vi "一体站流程自动启动.vi"(11 "参数":T1) -> ()   [LabVIEW 2016, in "PLC.lvlib"]
uses:
  PLC.lvlib
  <vilib>/ptbypt/NI_PtbyPt.lvlib
panel:
  out "s? t:f":enum16{"初始化", "采配水启动", "仪器操作", "反冲洗", "结束"}(ring)
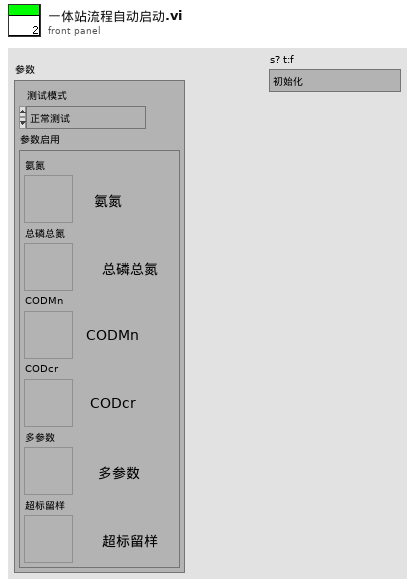
[diagram p1: front panel]
types:
  T1 = cluster{"测试模式":enum16{"正常测试", "集成干预"}, "参数启用":cluster{"氨氮":bool, "总磷总氮":bool, "CODMn":bool, "CODcr":bool, "多参数":bool, "超标留样":bool}}
  T2 = cluster{"命令":string, cluster{"starting address":u16, "holding register value":u16}}
  T3 = enum16{"启动测量", "标样核查", "零点核查", "跨度核查", "空白测试", "平行样测试", "加标回收", "空白校准", "标样校准", "初始化（清洗）", "停止测试", "仪器重启", "校时", "模式设置", "测量间隔设置"}
  T4 = cluster{"时间标识":timestamp, "设备":string, "日志信息":string, "流程参数":string}
  T5 = cluster{"测量模式":enum16{"水样测量", "标样核查", "零点核查", "跨度核查", "空白测试", "加标回收", "平行样", "校零", "校标"}}
  T6 = cluster{"时间标识":timestamp, "设备":string, "日志信息":string}
  T7 = enum16{"空闲", "水样测试", "标样核查", "零点核查", "跨度核查", "空白测试", "平行样测试", "加标回收", "空白校准", "标样校准", "初始化（清洗）"}
  T8 = enum32{"Bad", "Idle", "Run top level", "Running"}
  T9 = cluster{"R0":i16, "R1":i16, "R2":i16, "R3":i16, "R4":i16, "R5":i16, "R6":i16, "R7":i16, "R8":i16, "R9":i16, "R10":i16, "R11":i16, "R12":i16, "R13":i16, "R14":i16, "R15":i16, "R16":i16, "R17":i16, "R18":i16, "R19":i16, "R20":i16, "R21":i16, "R22":i16, "R23":i16, "R24":i16, "R25":i16, "R26":i16, "R27":i16, "R28":i16, "R29":i16, "R30":i16, "R31":i16, "R32":i16, "R33":i16, "R34":i16}
  T10 = cluster{"R100":i16, "R101":i16, "R102":i16, "R103":i16, "R104":i16, "R105":i16, "R106":i16, "R107":i16, "R108":i16, "R109":i16, "R110":i16, "R111":i16, "R112":i16, "R113":i16, "R114":i16, "R115":i16, "R116":i16, "R117":i16, "R118":i16, "R119":i16}
  T11 = cluster{"氨氮":bool, "总磷总氮":bool, "CODmn":bool, "CODCr":bool, "多参数":bool, "超标留样":bool}
  T12 = cluster{"因子编码":u32, "单位":u16, "标样参考值":sgl, "水样数据时间":timestamp, "水样实测值":sgl, "水样数据标识":string, "标样数据时间":timestamp, "标样实测值":sgl, "标样数据标识":string, "空白数据时间":timestamp, "空白实测值":sgl, "空白数据标识":string, "零点核查数据时间":timestamp, "零点核查实测值":sgl, "零点核查数据标识":string, "跨度核查数据时间":timestamp, "跨度核查实测值":sgl, "跨度核查数据标识":string, "加标回收数据时间":timestamp, "加标回收实测值":sgl, "加标回收数据标识":string, "平行样数据时间":timestamp, "平行样实测值":sgl, "平行样数据标识":string, "F0":sgl, "F1":sgl, "F2":sgl, "F3":sgl, "F4":sgl, "F5":sgl, "F6":sgl, "F7":sgl, "温度":sgl, "湿度":sgl, "X值":sgl, "fidrange":u16}
  T13 = cluster{"COD浓度（mg/L)":dbl, "水样启动时间":timestamp, "加标回收启动时间":timestamp, "CODMn工作状态":enum16{"空闲", "水样测试", "标样核查", "零点核查", "跨度核查", "空白测试", "平行样测试", "加标回收", "空白校准", "标样校准", "初始化（清洗）"}, "多列列表框":i32}
  T14 = cluster{"因子编码":u32, "单位":u16, "标样参考值":sgl, "水样数据时间":timestamp, "水样实测值":sgl, "水样数据标识":string, "标样数据时间":timestamp, "标样实测值":sgl, "标样数据标识":string, "空白数据时间":timestamp, "空白实测值":sgl, "空白数据标识":string, "零点核查数据时间":timestamp, "零点核查实测值":sgl, "零点核查数据标识":string, "跨度核查数据时间":timestamp, "跨度核查实测值":sgl, "跨度核查数据标识":string, "加标回收数据时间":timestamp, "加标回收实测值":sgl, "加标回收数据标识":string, "平行样数据时间":timestamp, "平行样实测值":sgl, "平行样数据标识":string}
  T15 = cluster{"氨氮":bool, "总磷总氮":bool, "CODMn":bool, "CODcr":bool, "多参数":bool, "超标留样":bool}
  T16 = cluster{"时间标识":timestamp, "参数":string, "数据类型":string, "集成干预测试浓度值":dbl, "集成干预前测试时间":timestamp, "集成干预前测试浓度值":dbl}
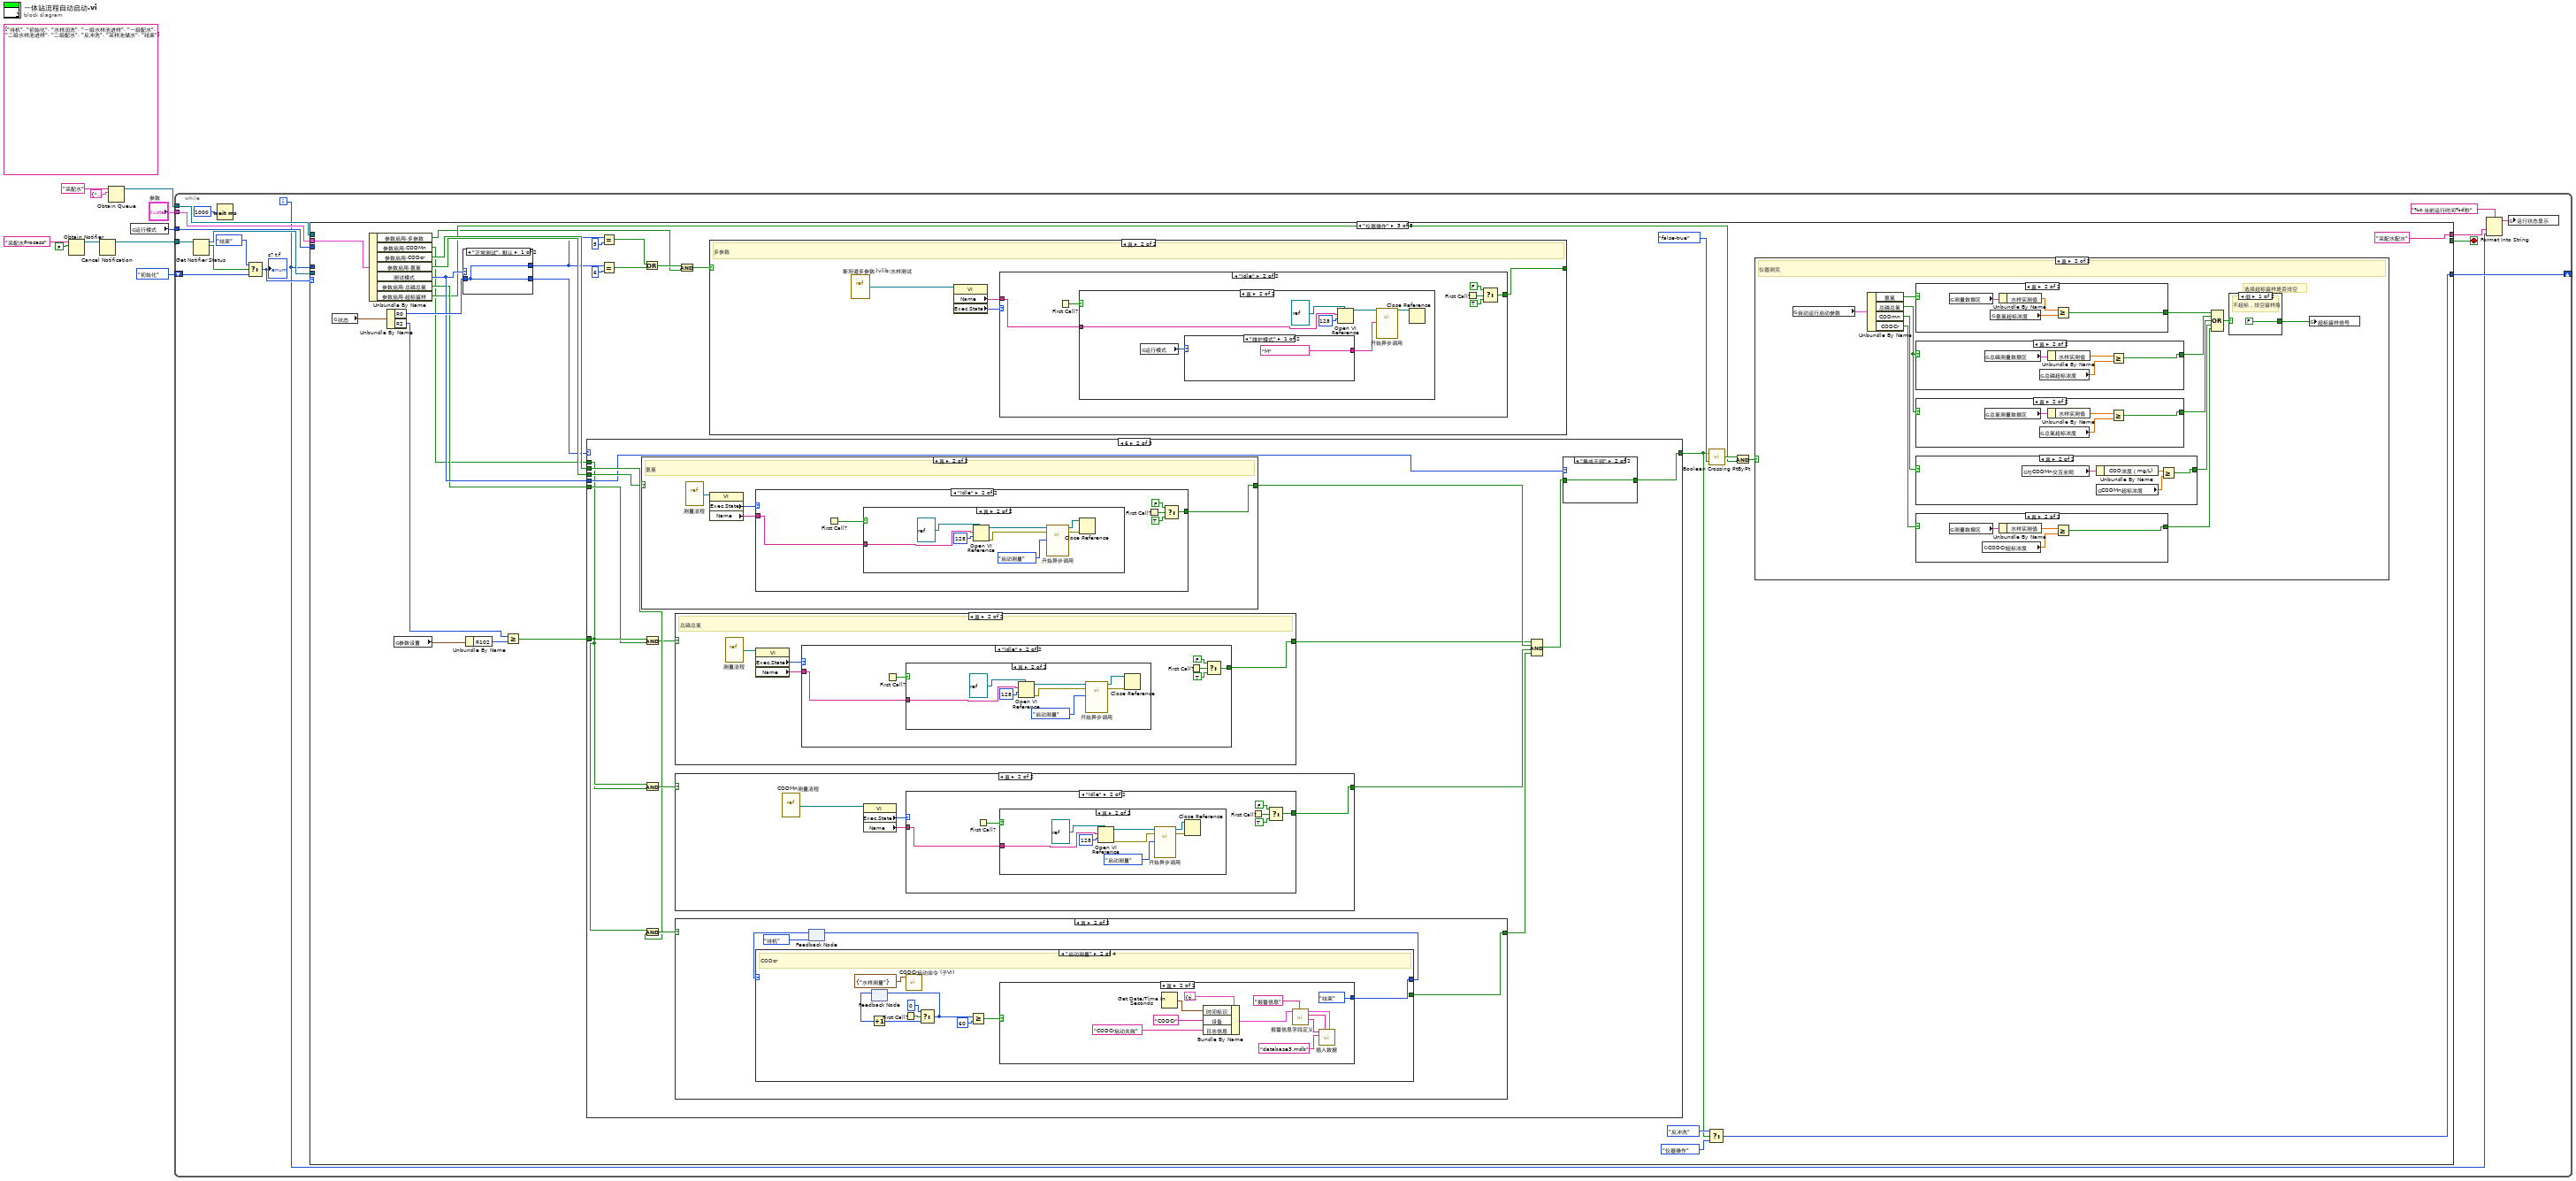
[diagram p0: block diagram]
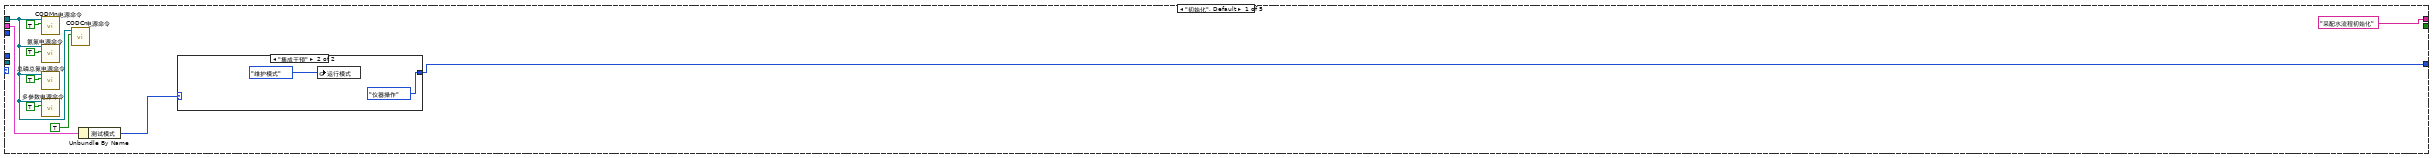
[diagram p2: hidden frame]
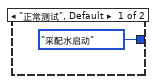
[diagram p3: hidden frame]
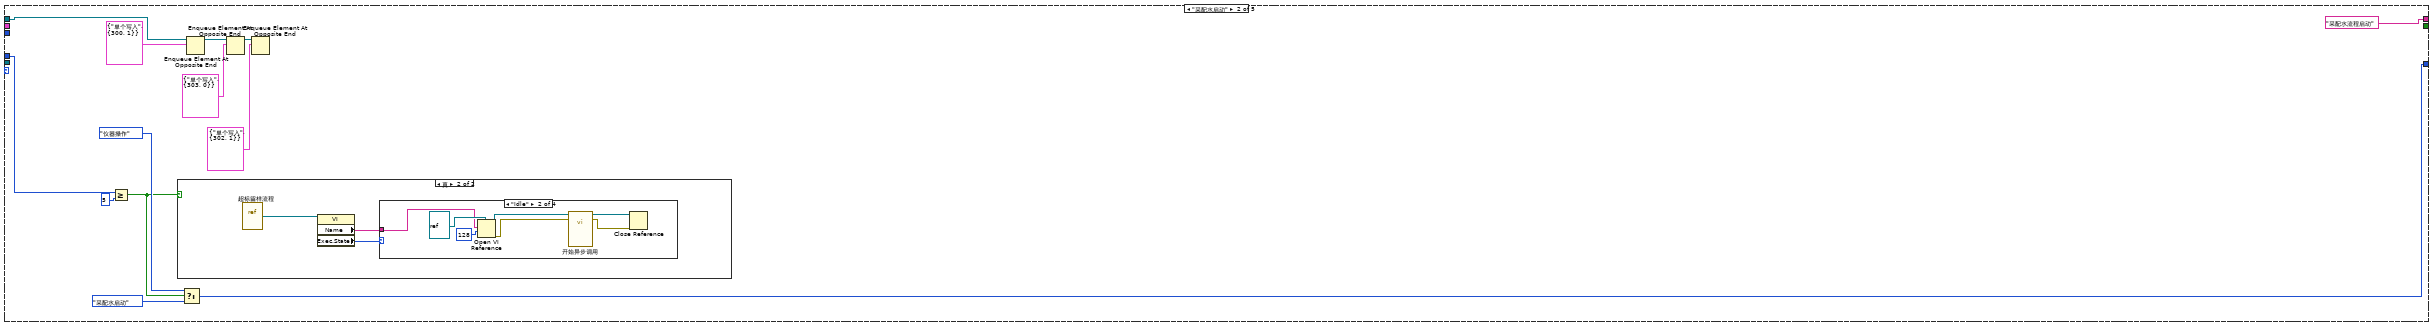
[diagram p4: hidden frame]
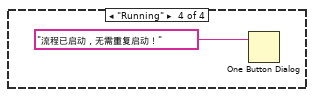
[diagram p8: hidden frame]
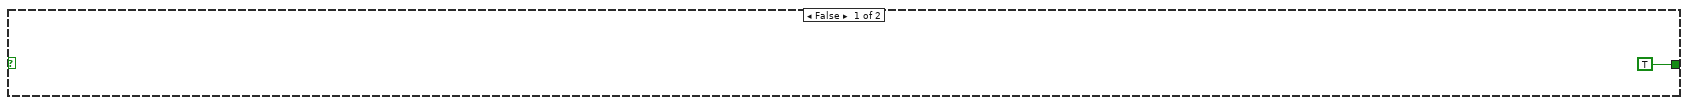
[diagram p9: hidden frame]
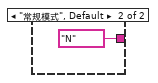
[diagram p12: hidden frame]
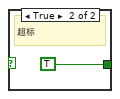
[diagram p14: hidden frame]
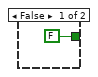
[diagram p15: hidden frame]
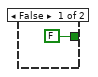
[diagram p16: hidden frame]
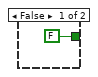
[diagram p17: hidden frame]
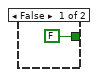
[diagram p18: hidden frame]
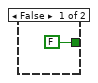
[diagram p19: hidden frame]
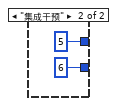
[diagram p20: hidden frame]
diagram:
  (unwired) string[][] [["待机"], ["初始化"], ["水样润洗"], ["一级水样池进样"], ["一级配水"], ["二级水样池进样"], ["二级配水"], ["反冲洗"], ["采样池储水"], ["结束"]] ("项名")
  n1 = Obtain Notifier(name (unnamed)="采配水Process" ("名称（未命名）"), notification data type=FALSE) -> (notifier out=w4:refnum<notifier>)  [unwired: 2 in, 2 out]
  n2 = Cancel Notification(0:w4) -> (8:w3:refnum<notifier>)  [unwired: 1 in, 2 out]
  n3 = Obtain Queue(name (unnamed)="采配水" ("名称（未命名）"), element data type=cluster{"命令":string, "数据":variant} {"命令"="", "数据"=variant}) -> (queue out=w7:refnum<queue>)  [unwired: 3 in, 2 out]
  n4 = global read "系统设置全局变量.vi" "运行模式"() -> (w1:enum16{"维护模式", "常规模式", "应急模式", "质控模式"})
  n5 = while {
    shift-right: [w23] -> _
    shift-left: enum16{"初始化", "采配水启动", "仪器操作", "反冲洗", "结束"}."初始化" ("枚举") -> [w19]
    tunnel: w7 -> [w26]
    tunnel: w3 -> [w22]
    tunnel: "参数" -> [w13]
    tunnel: w1 -> [w12]
    i -> [w11]
    stop <- w25 stop-if-true
    n6 = Get Notifier Status(notifier=w22) -> (notifier out=w14:refnum<notifier>, current notification=w21:bool)  [unwired: 1 in, 3 out]
    n7 = Wait (ms)(milliseconds to wait=u32 1000 ("等待时间（毫秒）")) -> ()  [unwired: 1 out]
    n8 = Select(t=enum16{"初始化", "采配水启动", "仪器操作", "反冲洗", "结束"}."结束" ("枚举"), s=w21, f=w19) -> (s? t:f=w18:enum16{"初始化", "采配水启动", "仪器操作", "反冲洗", "结束"})
    "s? t:f" <- w18
    n9 = case shown="\"仪器操作\"" w18 {
      tunnel: w26 -> [w31 w52 _ _ w475]
      tunnel: [_ _ _ _ TRUE] -> w25
      tunnel: [w30 w45 w89 w293 enum16{"初始化", "采配水启动", "仪器操作", "反冲洗", "结束"}."结束" ("枚举")] -> w23
      tunnel: ["采配水流程初始化" "采配水流程启动" "采配水配水" "等待测试完成" "采配水结束"] -> w15
      tunnel: w14 -> [_ _ _ _ w481]
      tunnel: w13 -> [w28 _ w91 w292 w478]
      tunnel: w12 -> [_ _ _ w289 w477]
      tunnel: w11 -> [_ w50 _ _ _]
      frame "初始化", Default {
        n10 = call "CODMn电源命令.vi"("通电/断电"=TRUE, "队列"=w31) -> ()  [unwired: 9 in, 1 out]
        n11 = call "氨氮电源命令.vi"("通电/断电"=TRUE, "队列"=w31) -> ()  [unwired: 9 in, 1 out]
        n12 = call "总磷总氮电源命令.vi"("通电/断电"=TRUE, "队列"=w31) -> ()  [unwired: 9 in, 1 out]
        n13 = call "多参数电源命令.vi"("通电/断电"=TRUE, "队列"=w31) -> ()  [unwired: 9 in, 1 out]
        n14 = call "CODCr电源命令.vi"("通电/断电"=TRUE, "队列"=w31) -> ()  [unwired: 9 in, 1 out]
        n15 = Unbundle By Name(w28) -> ("测试模式"=w27:enum16{"正常测试", "集成干预"})
        n16 = case shown="\"集成干预\"" w27 {
          tunnel: [enum16{"初始化", "采配水启动", "仪器操作", "反冲洗", "结束"}."采配水启动" ("枚举") enum16{"初始化", "采配水启动", "仪器操作", "反冲洗", "结束"}."仪器操作" ("枚举")] -> w30
          frame "正常测试", Default {
          }
          frame "集成干预" {
            n17 = global write "系统设置全局变量.vi" "运行模式"(enum16{"维护模式", "常规模式", "应急模式", "质控模式"}."维护模式" ("运行模式")) -> ()
          }
        }
      }
      frame "采配水启动" {
        n18 = Greater Or Equal?(x=w50, y=5) -> (x >= y?=w42:bool)
        n19 = case shown="真" w42 {
          frame False {
          }
          frame True {
            n20 = vi-ref "超标留样流程.vi"() -> (w55:refnum<vi>)
            n21 = property class="VI"(reference=w55) -> ("Name"=w54:string, "Exec.State"=w53:T8)  [unwired: 1 in, 2 out]
            n22 = case shown="\"Idle\"" w53 {
              tunnel: w54 -> [_ w58 _ _]
              frame "Bad", Default {
              }
              frame "Idle" {
                n23 = Open VI Reference(type specifier VI Refnum (for type only)=refnum<vi> refnum ("类型说明符VI引用句柄（仅用于类型）"), vi path=w58, options=128 ("选项")) -> (vi reference=w62:refnum<vi>, error out=w57:errorcluster)  [unwired: 3 in]
                n24 = call-by-ref "开始异步调用"(reference=w62, error in=w57) -> (reference out=w61:refnum<vi>, error out=w56:errorcluster)  [unwired: 12 in]
                n25 = Close Reference(reference=w61, error in (no error)=w56) -> ()  [unwired: 1 out]
              }
              frame "Run top level" {
              }
              frame "Running" {
                n26 = One Button Dialog(message="流程已启动，无需重复启动！" ("消息")) -> ()  [unwired: 1 in, 1 out]
              }
            }
          }
        }
        n27 = Select(t=enum16{"初始化", "采配水启动", "仪器操作", "反冲洗", "结束"}."仪器操作" ("枚举"), s=w42, f=enum16{"初始化", "采配水启动", "仪器操作", "反冲洗", "结束"}."采配水启动" ("枚举")) -> (s? t:f=w45:enum16{"初始化", "采配水启动", "仪器操作", "反冲洗", "结束"})
        n28 = Enqueue Element At Opposite End(queue=w52, element=T2 {"命令"="单个写入", {"starting address"=300, "holding register value"=1}} ("元素")) -> (queue out=w43:refnum<queue>)  [unwired: 2 in, 2 out]
        n29 = Enqueue Element At Opposite End(queue=w43, element=T2 {"命令"="单个写入", {"starting address"=303, "holding register value"=0}} ("元素")) -> (queue out=w40:refnum<queue>)  [unwired: 2 in, 2 out]
        n30 = Enqueue Element At Opposite End(queue=w40, element=T2 {"命令"="单个写入", {"starting address"=302, "holding register value"=1}} ("元素")) -> ()  [unwired: 2 in, 3 out]
      }
      frame "仪器操作" {
        n31 = global read "采配水全局变量.vi" "状态"() -> (w93:T9)
        n32 = Unbundle By Name(w91) -> ("参数启用.多参数"=w64:bool, "参数启用.CODMn"=w65:bool, "参数启用.CODcr"=w87:bool, "参数启用.氨氮"=w86:bool, "测试模式"=w79:enum16{"正常测试", "集成干预"}, "参数启用.总磷总氮"=w78:bool, "参数启用.超标留样"=w73:bool)
        n33 = Unbundle By Name(w93) -> ("R0"=w85:i16, "R2"=w80:i16)
        n34 = global read "采配水全局变量.vi" "参数设置"() -> (w82:T10)
        n35 = case shown="\"正常测试\", 默认" w79 {
          tunnel: w85 -> [w153 _]
          tunnel: [w153 i16 6 ("R0")] -> w84
          tunnel: [w153 i16 5 ("R0")] -> w70
          frame "正常测试", Default {
          }
          frame "集成干预" {
          }
        }
        n36 = Unbundle By Name(w82) -> ("R102"=w83:i16)
        n37 = Greater Or Equal?(x=w80, y=w83) -> (x >= y?=w81:bool)
        n38 = case shown="6" w84 {
          tunnel: [w157 w168 TRUE] -> w74
          tunnel: w87 -> [_ w175 _]
          tunnel: w86 -> [_ w174 _]
          tunnel: w81 -> [_ w167 _]
          tunnel: w79 -> [_ w170 _]
          tunnel: w78 -> [_ w166 _]
          tunnel: w65 -> [_ w163 _]
          frame 0, Default {
            n39 = global read "采配水全局变量.vi" "状态"() -> (w160:T9)
            n40 = global read "采配水全局变量.vi" "报警簇"() -> (w161:bool[])
            n41 = Unbundle By Name(w160) -> ("R0"=w159:i16)
            n42 = Equal To 0?(x=w159) -> (x = 0?=w162:bool)
            n43 = Index Array(array=w161, index=0 ("索引")) -> (element=w156:bool)
            n44 = Compound Arithmetic op=OR ("复合运算")(w162, w156) -> (w157:bool)
          }
          frame 6 {
            n45 = case "条件结构" shown="真" w174 {
              tunnel: [TRUE ("t") w199] -> w173
              frame False {
              }
              frame True {
                # "氨氮"
                n46 = vi-ref "测量流程.vi"() -> (w202:refnum<vi>)
                n47 = property class="VI"(reference=w202) -> ("Exec.State"=w201:T8, "Name"=w200:string)  [unwired: 1 in, 2 out]
                n48 = case shown="\"Idle\"" w201 {
                  tunnel: w200 -> [_ w208]
                  tunnel: [_ w203] -> w199
                  frame "Bad", Default {
                  }
                  frame "Idle" {
                    n49 = First Call?() -> (First Call?: T/F=w207:bool)
                    n50 = case shown="真" w207 {
                      tunnel: w208 -> [_ w213]
                      frame False {
                      }
                      frame True {
                        n51 = Open VI Reference(type specifier VI Refnum (for type only)=refnum<vi> refnum, vi path=w213, options=128 ("选项")) -> (vi reference=w211:refnum<vi>, error out=w214:errorcluster)  [unwired: 3 in]
                        n52 = call-by-ref "开始异步调用"(reference=w211, error in=w214, "控制命令"=T3."启动测量") -> (reference out=w215:refnum<vi>, error out=w216:errorcluster)  [unwired: 11 in]
                        n53 = Close Reference(reference=w215, error in (no error)=w216) -> ()  [unwired: 1 out]
                      }
                    }
                    n54 = First Call?() -> (First Call?: T/F=w206:bool)
                    n55 = Select(t=FALSE, s=w206, f=TRUE) -> (s? t:f=w203:bool)
                  }
                }
              }
            }
            n56 = And(x=w167, y=w166) -> (x .and. y?=w165:bool)
            n57 = And(x=w167, y=w163) -> (x .and. y?=w177:bool)
            n58 = And(x=w167, y=w175) -> (x .and. y?=w176:bool)
            n59 = case "条件结构" shown="真" w165 {
              tunnel: [TRUE ("t") w179] -> w164
              frame False {
              }
              frame True {
                # "总磷总氮"
                n60 = vi-ref "测量流程.vi"() -> (w182:refnum<vi>)
                n61 = property class="VI"(reference=w182) -> ("Exec.State"=w181:T8, "Name"=w180:string)  [unwired: 1 in, 2 out]
                n62 = case shown="\"Idle\"" w181 {
                  tunnel: w180 -> [_ w188]
                  tunnel: [_ w183] -> w179
                  frame "Bad", Default {
                  }
                  frame "Idle" {
                    n63 = First Call?() -> (First Call?: T/F=w187:bool)
                    n64 = case shown="真" w187 {
                      tunnel: w188 -> [_ w193]
                      frame False {
                      }
                      frame True {
                        n65 = Open VI Reference(type specifier VI Refnum (for type only)=refnum<vi> refnum, vi path=w193, options=128 ("选项")) -> (vi reference=w191:refnum<vi>, error out=w194:errorcluster)  [unwired: 3 in]
                        n66 = call-by-ref "开始异步调用"(reference=w191, error in=w194, "控制命令"=T3."启动测量") -> (reference out=w195:refnum<vi>, error out=w196:errorcluster)  [unwired: 11 in]
                        n67 = Close Reference(reference=w195, error in (no error)=w196) -> ()  [unwired: 1 out]
                      }
                    }
                    n68 = First Call?() -> (First Call?: T/F=w186:bool)
                    n69 = Select(t=FALSE, s=w186, f=TRUE) -> (s? t:f=w183:bool)
                  }
                }
              }
            }
            n70 = case shown="真" w177 {
              tunnel: [TRUE w270] -> w172
              frame False {
              }
              frame True {
                n71 = vi-ref "CODMn测量流程.vi"() -> (w271:refnum<vi>)
                n72 = property class="VI"(reference=w271) -> ("Exec.State"=w272:T8, "Name"=w273:string)  [unwired: 1 in, 2 out]
                n73 = case shown="\"Idle\"" w272 {
                  tunnel: w273 -> [_ w279]
                  tunnel: [_ w274] -> w270
                  frame "Bad", Default {
                  }
                  frame "Idle" {
                    n74 = First Call?() -> (First Call?: T/F=w278:bool)
                    n75 = case shown="真" w278 {
                      tunnel: w279 -> [_ w284]
                      frame False {
                      }
                      frame True {
                        n76 = Open VI Reference(type specifier VI Refnum (for type only)=refnum<vi> refnum, vi path=w284, options=128 ("选项")) -> (vi reference=w282:refnum<vi>, error out=w285:errorcluster)  [unwired: 3 in]
                        n77 = call-by-ref "开始异步调用"(reference=w282, error in=w285, "控制命令"=T3."启动测量") -> (reference out=w286:refnum<vi>, error out=w287:errorcluster)  [unwired: 11 in]
                        n78 = Close Reference(reference=w286, error in (no error)=w287) -> ()  [unwired: 1 out]
                      }
                    }
                    n79 = First Call?() -> (First Call?: T/F=w277:bool)
                    n80 = Select(t=FALSE, s=w277, f=TRUE) -> (s? t:f=w274:bool)
                  }
                }
              }
            }
            n81 = case shown="真" w176 {
              tunnel: [TRUE w218] -> w171
              frame False {
              }
              frame True {
                n82 = feedback #1(enum16{"待机", "启动测量", "测量中", "结束"}."待机") -> (w220:enum16{"待机", "启动测量", "测量中", "结束"})
                n83 = case shown="\"启动测量\"" w220 {
                  tunnel: [enum16{"待机", "启动测量", "测量中", "结束"}."启动测量" w236 w256 enum16{"待机", "启动测量", "测量中", "结束"}."结束"] -> w219
                  tunnel: [_ _ _ TRUE] -> w218
                  frame "待机", Default {
                    n84 = Get Date/Time In Seconds() -> (seconds since 1Jan1904=w226:timestamp)
                    n85 = Bundle By Name(cluster=T4 {"时间标识"=timestamp(0 s since 1904-01-01), "设备"="", "日志信息"="", "流程参数"=""} ("data in"), "时间标识"=w226, "设备"="CODCr", "日志信息"="-->>CODCr启动") -> (w222:T4)
                    n86 = call "总磷总氮操作日志.vi"("data in"=w222) -> ()  [unwired: 11 in]
                  }
                  frame "启动测量" {
                    # "CODcr"
                    n87 = feedback #2() -> (w232:i32)  [unwired: 1 in]
                    n88 = Increment(x=w232) -> (x+1=w233:i32)
                    n89 = First Call?() -> (First Call?: T/F=w231:bool)
                    n90 = call "CODCr启动命令 (子VI).vi"("启动测量模式"=T5 {"测量模式"=enum."水样测量"}) -> ()  [unwired: 11 in]
                    n91 = Select(t=0, s=w231, f=w233) -> (s? t:f=w234:i32)
                    n92 = feedback-in #2(w234) -> ()
                    n93 = Greater Or Equal?(x=w234, y=60) -> (x >= y?=w229:bool)
                    n94 = case shown="真" w229 {
                      tunnel: [w237 enum16{"待机", "启动测量", "测量中", "结束"}."结束"] -> w236
                      frame False {
                        n95 = global read "CODcr全局变量.vi" "工作状态"() -> (w238:T7)
                        n96 = Not Equal To 0?(x=w238) -> (x != 0?=w239:bool)
                        n97 = Select(t=enum16{"待机", "启动测量", "测量中", "结束"}."测量中", s=w239, f=enum16{"待机", "启动测量", "测量中", "结束"}."启动测量") -> (s? t:f=w237:enum16{"待机", "启动测量", "测量中", "结束"})
                      }
                      frame True {
                        n98 = Get Date/Time In Seconds() -> (seconds since 1Jan1904=w248:timestamp)
                        n99 = Bundle By Name(cluster=T6 {"时间标识"=timestamp(0 s since 1904-01-01), "设备"="", "日志信息"=""} ("data in"), "时间标识"=w248, "设备"="CODCr", "日志信息"="CODCr启动失败") -> (w242:T6)
                        n100 = call "报警信息字段定义.vi"("table输入"="报警信息", "data in"=w242) -> ("table输出"=w245:string, "columns"=w246:string[], "data out"=w247:T6)  [unwired: 7 in]
                        n101 = call "插入数据.vi"("data"=w247, "columns"=w246, "database"="database3.mdb", "table"=w245) -> ()  [unwired: 7 in, 1 out]
                      }
                    }
                  }
                  frame "测量中" {
                    n102 = global read "CODcr全局变量.vi" "工作状态"() -> (w255:T7)
                    n103 = Equal?(x=w255, y=T7."空闲" ("工作状态")) -> (x = y?=w254:bool)
                    n104 = case shown="假" w254 {
                      tunnel: [w257 enum16{"待机", "启动测量", "测量中", "结束"}."结束"] -> w256
                      frame False {
                        n105 = flat-sequence {
                          tunnel: [enum16{"待机", "启动测量", "测量中", "结束"}."测量中"] -> w257
                          frame #0 {
                            n106 = Wait (ms)(milliseconds to wait=u32 1000 ("等待时间（毫秒）")) -> ()  [unwired: 1 out]
                          }
                          frame #1 {
                          }
                        }
                      }
                      frame True {
                      }
                    }
                  }
                  frame "结束" {
                    n107 = First Call?() -> (First Call?: T/F=w261:bool)
                    n108 = case shown="真" w261 {
                      frame False {
                      }
                      frame True {
                        n109 = Get Date/Time In Seconds() -> (seconds since 1Jan1904=w268:timestamp)
                        n110 = Bundle By Name(cluster=T4 {"时间标识"=timestamp(0 s since 1904-01-01), "设备"="", "日志信息"="", "流程参数"=""} ("data in"), "时间标识"=w268, "设备"="CODCr", "日志信息"="-->>CODCr停止") -> (w264:T4)
                        n111 = call "总磷总氮操作日志.vi"("data in"=w264) -> ()  [unwired: 11 in]
                      }
                    }
                  }
                }
                n112 = feedback-in #1(w219) -> ()
              }
            }
            n113 = Compound Arithmetic op=AND ("复合运算")(w164, w173, w172, w171) -> (w169:bool)
            n114 = case shown="\"集成干预\"" w170 {
              tunnel: w169 -> [_ w197]
              tunnel: [_ w197] -> w168
              frame "正常测试", Default {
              }
              frame "集成干预" {
              }
            }
          }
          frame 7..9 {
          }
        }
        n115 = Equal?(x=w70, y=i16 5) -> (x = y?=w71:bool)
        n116 = Equal?(x=w70, y=i16 6) -> (x = y?=w67:bool)
        n117 = Or(x=w71, y=w67) -> (x .or. y?=w68:bool)
        n118 = And(x=w68, y=w64) -> (x .and. y?=w66:bool)
        n119 = case shown="真" w66 {
          tunnel: [TRUE ("t") w95] -> _
          frame False {
          }
          frame True {
            # "多参数"
            n120 = vi-ref "斯坦道多参数.lvlib:水样测试.vi"() -> (w97:refnum<vi>)
            n121 = property class="VI"(reference=w97) -> ("Name"=w96:string, "Exec.State"=w98:T8)  [unwired: 1 in, 2 out]
            n122 = case shown="\"Idle\"" w98 {
              tunnel: w96 -> [_ w104]
              tunnel: [_ w99] -> w95
              frame "Bad", Default {
              }
              frame "Idle" {
                n123 = First Call?() -> (First Call?: T/F=w103:bool)
                n124 = case shown="真" w103 {
                  tunnel: w104 -> [_ w110]
                  frame False {
                  }
                  frame True {
                    n125 = global read "系统设置全局变量.vi" "运行模式"() -> (w107:enum16{"维护模式", "常规模式", "应急模式", "质控模式"})
                    n126 = case shown="\"维护模式\"" w107 {
                      tunnel: ["M" ("数据标记表") "N" ("数据标记表")] -> w106
                      frame "维护模式" {
                      }
                      frame "常规模式", Default {
                      }
                    }
                    n127 = Open VI Reference(type specifier VI Refnum (for type only)=refnum<vi> refnum, vi path=w110, options=128 ("选项")) -> (vi reference=w109:refnum<vi>)  [unwired: 3 in, 1 out]
                    n128 = call-by-ref "开始异步调用"(reference=w109, "数据标记表"=w106) -> (reference out=w108:refnum<vi>)  [unwired: 12 in, 1 out]
                    n129 = Close Reference(reference=w108) -> ()  [unwired: 1 in, 1 out]
                  }
                }
                n130 = First Call?() -> (First Call?: T/F=w102:bool)
                n131 = Select(t=FALSE, s=w102, f=TRUE) -> (s? t:f=w99:bool)
              }
            }
          }
        }
        n132 = Select(t=enum16{"初始化", "采配水启动", "仪器操作", "反冲洗", "结束"}."反冲洗" ("枚举"), s=w74, f=enum16{"初始化", "采配水启动", "仪器操作", "反冲洗", "结束"}."仪器操作" ("枚举")) -> (s? t:f=w89:enum16{"初始化", "采配水启动", "仪器操作", "反冲洗", "结束"})
        n133 = call <vilib>:"Boolean Crossing PtByPt.vi"("direction"=enum16{"either", "false-true", "true-false"}."false-true", "input"=w74) -> ("crossing"=w76:bool)  [unwired: 1 in]
        n134 = And(x=w76, y=w73) -> (x .and. y?=w75:bool)
        n135 = case shown="真" w75 {
          frame False {
          }
          frame True {
            # "选择超标留样是否排空"
            # "仪器测完"
            n136 = global read "系统设置全局变量.vi" "自动运行启动参数"() -> (w118:T11)
            n137 = Unbundle By Name(w118) -> ("氨氮"=w117:bool, "总磷总氮"=w116:bool, "CODmn"=w115:bool, "CODCr"=w114:bool)
            n138 = case shown="真" w117 {
              tunnel: [FALSE w151] -> w125
              frame False {
              }
              frame True {
                n139 = global read "VAR总磷总氮全局变量.vi" "测量数据区"() -> (w150:T12)
                n140 = global read "外部交互全局.vi" "氨氮超标浓度"() -> (w149:dbl)
                n141 = Unbundle By Name(w150) -> ("水样实测值"=w152:sgl)
                n142 = Greater Or Equal?(x=w152, y=w149) -> (x >= y?=w151:bool)
              }
            }
            n143 = case shown="真" w116 {
              tunnel: [FALSE w147] -> w124
              frame False {
              }
              frame True {
                n144 = global read "VAR总磷总氮全局变量.vi" "总磷测量数据区"() -> (w144:T12)
                n145 = global read "外部交互全局.vi" "总磷超标浓度"() -> (w145:dbl)
                n146 = Unbundle By Name(w144) -> ("水样实测值"=w146:sgl)
                n147 = Greater Or Equal?(x=w146, y=w145) -> (x >= y?=w147:bool)
              }
            }
            n148 = case shown="真" w116 {
              tunnel: [FALSE w142] -> w123
              frame False {
              }
              frame True {
                n149 = global read "VAR总磷总氮全局变量.vi" "总氮测量数据区"() -> (w139:T12)
                n150 = global read "外部交互全局.vi" "总氮超标浓度"() -> (w140:dbl)
                n151 = Unbundle By Name(w139) -> ("水样实测值"=w141:sgl)
                n152 = Greater Or Equal?(x=w141, y=w140) -> (x >= y?=w142:bool)
              }
            }
            n153 = case shown="真" w115 {
              tunnel: [FALSE w137] -> w122
              frame False {
              }
              frame True {
                n154 = global read "modbus slave全局.vi" "与CODMn交互全局"() -> (w135:T13)
                n155 = Unbundle By Name(w135) -> ("COD浓度（mg/L)"=w134:dbl)
                n156 = global read "外部交互全局.vi" "CODMn超标浓度"() -> (w136:dbl)
                n157 = Greater Or Equal?(x=w134, y=w136) -> (x >= y?=w137:bool)
              }
            }
            n158 = case shown="真" w114 {
              tunnel: [FALSE w132] -> w121
              frame False {
              }
              frame True {
                n159 = global read "CODcr全局变量.vi" "测量数据区"() -> (w129:T14)
                n160 = global read "外部交互全局.vi" "CODCr超标浓度"() -> (w130:dbl)
                n161 = Unbundle By Name(w129) -> ("水样实测值"=w131:sgl)
                n162 = Greater Or Equal?(x=w131, y=w130) -> (x >= y?=w132:bool)
              }
            }
            n163 = Compound Arithmetic op=OR ("复合运算")(w125, w124, w123, w122, w121) -> (w120:bool)
            n164 = case shown="假" w120 {
              tunnel: [FALSE ("超标留样信号") TRUE ("超标留样信号")] -> w119
              frame False {
                # "不超标，排空留样瓶"
              }
              frame True {
                # "超标"
              }
            }
            n165 = global write "外部交互全局.vi" "超标留样信号"(w119) -> ()
          }
        }
      }
      frame "反冲洗" {
        n166 = First Call?() -> (First Call?: T/F=w290:bool)
        n167 = case shown="真" w290 {
          tunnel: w292 -> [_ w302]
          tunnel: w289 -> [_ w299]
          frame False {
          }
          frame True {
            n168 = Unbundle By Name(w302) -> ("测试模式"=w301:enum16{"正常测试", "集成干预"}, "参数启用"=w300:T15)
            n169 = case shown="\"正常测试\", 默认" w301 {
              tunnel: w300 -> [w311 w398]
              tunnel: w299 -> [_ w392]
              frame "正常测试", Default {
                n170 = global read "系统设置全局变量.vi" "运行模式"() -> (w309:enum16{"维护模式", "常规模式", "应急模式", "质控模式"})
                n171 = global read "采配水全局变量.vi" "输入状态"() -> (w308:bool[])
                n172 = global read "采配水全局变量.vi" "报警簇"() -> (w316:bool[])
                n173 = case shown="\"维护模式\"" w309 {
                  tunnel: ["M" ("table") "N" ("table")] -> w310
                  frame "维护模式" {
                  }
                  frame "常规模式", Default {
                  }
                }
                n174 = Index Array(array=w308, index=7 ("索引")) -> (element=w306:bool)
                n175 = Index Array(array=w316, index #1=0 ("索引"), index #2=11 ("索引")) -> (element #1=w313:bool, element #2=w312:bool)
                n176 = Select(t="P" ("数据标识"), s=w306, f="Z" ("数据标识")) -> (s? t:f=w303:string)
                n177 = case shown="真" w313 {
                  tunnel: w312 -> [w322 _]
                  tunnel: w311 -> [w321 w336]
                  tunnel: w310 -> [w319 w330]
                  tunnel: w303 -> [_ w329]
                  frame False {
                    n178 = Unbundle By Name(w321) -> ("氨氮"=w320:bool)
                    n179 = case shown="真" w322 {
                      tunnel: w320 -> [_ w324]
                      tunnel: w319 -> [_ w323]
                      frame False {
                      }
                      frame True {
                        n180 = case shown="真" w324 {
                          tunnel: w323 -> [_ w325]
                          tunnel: [_ w326] -> _
                          frame False {
                          }
                          frame True {
                            n181 = call "取水点无水样数据存储.vi"("数据标识"="lw", "数据类型"=w325, "table"="氨氮") -> ("error out"=w326:errorcluster)  [unwired: 8 in]
                          }
                        }
                      }
                    }
                  }
                  frame True {
                    n182 = Unbundle By Name(w336) -> ("氨氮"=w335:bool, "CODMn"=w334:bool, "CODcr"=w333:bool, "多参数"=w332:bool, "总磷总氮"=w331:bool)
                    n183 = case shown="真" w335 {
                      tunnel: w330 -> [_ w389]
                      tunnel: [_ w390] -> _
                      tunnel: w329 -> [_ w388]
                      frame False {
                      }
                      frame True {
                        n184 = call "取水点无水样数据存储.vi"("数据标识"=w388, "数据类型"=w389, "table"="氨氮") -> ("error out"=w390:errorcluster)  [unwired: 8 in]
                      }
                    }
                    n185 = case shown="真" w334 {
                      tunnel: w330 -> [_ w386]
                      tunnel: [_ w385] -> _
                      tunnel: w329 -> [_ w384]
                      frame False {
                      }
                      frame True {
                        n186 = call "取水点无水样数据存储.vi"("数据标识"=w384, "数据类型"=w386, "table"="CODMn") -> ("error out"=w385:errorcluster)  [unwired: 8 in]
                      }
                    }
                    n187 = case shown="真" w333 {
                      tunnel: w330 -> [_ w382]
                      tunnel: [_ w381] -> _
                      tunnel: w329 -> [_ w380]
                      frame False {
                      }
                      frame True {
                        n188 = call "取水点无水样数据存储.vi"("数据标识"=w380, "数据类型"=w382, "table"="CODCr") -> ("error out"=w381:errorcluster)  [unwired: 8 in]
                      }
                    }
                    n189 = case shown="真" w331 {
                      tunnel: w330 -> [_ w337]
                      tunnel: [_ w339] -> _
                      tunnel: w329 -> [_ w338]
                      frame False {
                      }
                      frame True {
                        n190 = call "取水点无水样数据存储.vi"("数据标识"=w338, "数据类型"=w337, "table"="总氮") -> ("error out"=w340:errorcluster)  [unwired: 8 in]
                        n191 = call "取水点无水样数据存储.vi"("error in (no error)"=w340, "数据标识"=w337, "数据类型"=w337, "table"="总磷") -> ("error out"=w339:errorcluster)  [unwired: 7 in]
                      }
                    }
                    n192 = case shown="真" w332 {
                      tunnel: w330 -> [_ w351]
                      tunnel: w329 -> [_ w343]
                      frame False {
                      }
                      frame True {
                        n193 = global read "断电保存变量.vi" "Cond"() -> (w346:bool)
                        n194 = global read "断电保存变量.vi" "Turb"() -> (w347:bool)
                        n195 = global read "断电保存变量.vi" "DO"() -> (w348:bool)
                        n196 = global read "断电保存变量.vi" "pH"() -> (w349:bool)
                        n197 = case shown="真" w349 {
                          tunnel: w351 -> [_ w374]
                          tunnel: [_ w373] -> _
                          tunnel: w343 -> [_ w372]
                          frame False {
                          }
                          frame True {
                            n198 = call "取水点无水样数据存储.vi"("数据标识"=w372, "数据类型"=w374, "table"="pH") -> ("error out"=w373:errorcluster)  [unwired: 8 in]
                          }
                        }
                        n199 = case shown="真" w348 {
                          tunnel: w351 -> [_ w370]
                          tunnel: [_ w369] -> _
                          tunnel: w343 -> [_ w368]
                          frame False {
                          }
                          frame True {
                            n200 = call "取水点无水样数据存储.vi"("数据标识"=w368, "数据类型"=w370, "table"="DO") -> ("error out"=w369:errorcluster)  [unwired: 8 in]
                          }
                        }
                        n201 = case shown="真" w347 {
                          tunnel: w351 -> [_ w362]
                          tunnel: [_ w361] -> _
                          tunnel: w343 -> [_ w360]
                          frame False {
                          }
                          frame True {
                            n202 = call "取水点无水样数据存储.vi"("数据标识"=w360, "数据类型"=w362, "table"="浊度") -> ("error out"=w361:errorcluster)  [unwired: 8 in]
                          }
                        }
                        n203 = case shown="真" w346 {
                          tunnel: w351 -> [_ w366]
                          tunnel: [_ w365] -> _
                          tunnel: w343 -> [_ w364]
                          frame False {
                          }
                          frame True {
                            n204 = call "取水点无水样数据存储.vi"("数据标识"=w364, "数据类型"=w366, "table"="电导率") -> ("error out"=w365:errorcluster)  [unwired: 8 in]
                          }
                        }
                        n205 = global read "断电保存变量.vi" "藻密度"() -> (w344:bool)
                        n206 = global read "断电保存变量.vi" "Temp"() -> (w350:bool)
                        n207 = global read "断电保存变量.vi" "叶绿素a启用"() -> (w345:bool)
                        n208 = case shown="真" w344 {
                          tunnel: w351 -> [_ w354]
                          tunnel: [_ w353] -> _
                          tunnel: w343 -> [_ w352]
                          frame False {
                          }
                          frame True {
                            n209 = call "取水点无水样数据存储.vi"("数据标识"=w352, "数据类型"=w354, "table"="藻密度") -> ("error out"=w353:errorcluster)  [unwired: 8 in]
                          }
                        }
                        n210 = case shown="真" w350 {
                          tunnel: w351 -> [_ w378]
                          tunnel: [_ w377] -> _
                          tunnel: w343 -> [_ w376]
                          frame False {
                          }
                          frame True {
                            n211 = call "取水点无水样数据存储.vi"("数据标识"=w376, "数据类型"=w378, "table"="水温") -> ("error out"=w377:errorcluster)  [unwired: 8 in]
                          }
                        }
                        n212 = case shown="真" w345 {
                          tunnel: w351 -> [_ w358]
                          tunnel: [_ w357] -> _
                          tunnel: w343 -> [_ w356]
                          frame False {
                          }
                          frame True {
                            n213 = call "取水点无水样数据存储.vi"("数据标识"=w356, "数据类型"=w358, "table"="叶绿素a") -> ("error out"=w357:errorcluster)  [unwired: 8 in]
                          }
                        }
                      }
                    }
                  }
                }
              }
              frame "集成干预" {
                n214 = Unbundle By Name(w398) -> ("氨氮"=w397:bool, "CODMn"=w396:bool, "CODcr"=w395:bool, "多参数"=w394:bool, "总磷总氮"=w393:bool)
                n215 = case shown="真" w397 {
                  tunnel: w392 -> [_ w470]
                  frame False {
                  }
                  frame True {
                    n216 = call "获取最近两组水样测试数据.vi"("运行模式"=w470, "table"="氨氮") -> ("error out"=w471:errorcluster, "存储变量"=w472:T16)  [unwired: 8 in]
                    n217 = call "集成干预测试数据存储.vi"("error in (no error)"=w471, "存储变量"=w472) -> ()  [unwired: 9 in, 1 out]
                  }
                }
                n218 = case shown="真" w396 {
                  tunnel: w392 -> [_ w466]
                  frame False {
                  }
                  frame True {
                    n219 = call "获取最近两组水样测试数据.vi"("运行模式"=w466, "table"="CODMn") -> ("error out"=w467:errorcluster, "存储变量"=w468:T16)  [unwired: 8 in]
                    n220 = call "集成干预测试数据存储.vi"("error in (no error)"=w467, "存储变量"=w468) -> ()  [unwired: 9 in, 1 out]
                  }
                }
                n221 = case shown="真" w395 {
                  tunnel: w392 -> [_ w462]
                  frame False {
                  }
                  frame True {
                    n222 = call "获取最近两组水样测试数据.vi"("运行模式"=w462, "table"="CODCr") -> ("error out"=w463:errorcluster, "存储变量"=w464:T16)  [unwired: 8 in]
                    n223 = call "集成干预测试数据存储.vi"("error in (no error)"=w463, "存储变量"=w464) -> ()  [unwired: 9 in, 1 out]
                  }
                }
                n224 = case shown="真" w393 {
                  tunnel: w392 -> [_ w399]
                  frame False {
                  }
                  frame True {
                    n225 = call "获取最近两组水样测试数据.vi"("运行模式"=w399, "table"="总磷") -> ("error out"=w404:errorcluster, "存储变量"=w405:T16)  [unwired: 8 in]
                    n226 = call "集成干预测试数据存储.vi"("error in (no error)"=w404, "存储变量"=w405) -> ("error out"=w400:errorcluster)  [unwired: 9 in]
                    n227 = call "获取最近两组水样测试数据.vi"("error in (no error)"=w400, "运行模式"=w399, "table"="总氮") -> ("error out"=w403:errorcluster, "存储变量"=w402:T16)  [unwired: 7 in]
                    n228 = call "集成干预测试数据存储.vi"("error in (no error)"=w403, "存储变量"=w402) -> ()  [unwired: 9 in, 1 out]
                  }
                }
                n229 = case shown="真" w394 {
                  tunnel: w392 -> [_ w407]
                  frame False {
                  }
                  frame True {
                    n230 = global read "断电保存变量.vi" "Temp"() -> (w414:bool)
                    n231 = case shown="真" w414 {
                      tunnel: [_ w458] -> w420
                      tunnel: w407 -> [_ w457]
                      frame False {
                      }
                      frame True {
                        n232 = call "获取最近两组水样测试数据.vi"("运行模式"=w457, "table"="水温") -> ("error out"=w461:errorcluster, "存储变量"=w460:T16)  [unwired: 8 in]
                        n233 = call "集成干预测试数据存储.vi"("error in (no error)"=w461, "存储变量"=w460) -> ("error out"=w458:errorcluster)  [unwired: 9 in]
                      }
                    }
                    n234 = global read "断电保存变量.vi" "pH"() -> (w413:bool)
                    n235 = case shown="真" w413 {
                      tunnel: [_ w453] -> w419
                      tunnel: w420 -> [_ w452]
                      tunnel: w407 -> [_ w451]
                      frame False {
                      }
                      frame True {
                        n236 = call "获取最近两组水样测试数据.vi"("error in (no error)"=w452, "运行模式"=w451, "table"="pH") -> ("error out"=w456:errorcluster, "存储变量"=w455:T16)  [unwired: 7 in]
                        n237 = call "集成干预测试数据存储.vi"("error in (no error)"=w456, "存储变量"=w455) -> ("error out"=w453:errorcluster)  [unwired: 9 in]
                      }
                    }
                    n238 = global read "断电保存变量.vi" "DO"() -> (w412:bool)
                    n239 = case shown="真" w412 {
                      tunnel: [_ w447] -> w418
                      tunnel: w419 -> [_ w446]
                      tunnel: w407 -> [_ w445]
                      frame False {
                      }
                      frame True {
                        n240 = call "获取最近两组水样测试数据.vi"("error in (no error)"=w446, "运行模式"=w445, "table"="DO") -> ("error out"=w450:errorcluster, "存储变量"=w449:T16)  [unwired: 7 in]
                        n241 = call "集成干预测试数据存储.vi"("error in (no error)"=w450, "存储变量"=w449) -> ("error out"=w447:errorcluster)  [unwired: 9 in]
                      }
                    }
                    n242 = global read "断电保存变量.vi" "Cond"() -> (w411:bool)
                    n243 = case shown="真" w411 {
                      tunnel: [_ w441] -> w417
                      tunnel: w418 -> [_ w440]
                      tunnel: w407 -> [_ w439]
                      frame False {
                      }
                      frame True {
                        n244 = call "获取最近两组水样测试数据.vi"("error in (no error)"=w440, "运行模式"=w439, "table"="电导率") -> ("error out"=w444:errorcluster, "存储变量"=w443:T16)  [unwired: 7 in]
                        n245 = call "集成干预测试数据存储.vi"("error in (no error)"=w444, "存储变量"=w443) -> ("error out"=w441:errorcluster)  [unwired: 9 in]
                      }
                    }
                    n246 = global read "断电保存变量.vi" "Turb"() -> (w410:bool)
                    n247 = case shown="真" w410 {
                      tunnel: [_ w435] -> w416
                      tunnel: w417 -> [_ w434]
                      tunnel: w407 -> [_ w433]
                      frame False {
                      }
                      frame True {
                        n248 = call "获取最近两组水样测试数据.vi"("error in (no error)"=w434, "运行模式"=w433, "table"="浊度") -> ("error out"=w438:errorcluster, "存储变量"=w437:T16)  [unwired: 7 in]
                        n249 = call "集成干预测试数据存储.vi"("error in (no error)"=w438, "存储变量"=w437) -> ("error out"=w435:errorcluster)  [unwired: 9 in]
                      }
                    }
                    n250 = global read "断电保存变量.vi" "叶绿素a启用"() -> (w409:bool)
                    n251 = case shown="真" w409 {
                      tunnel: [_ w429] -> w415
                      tunnel: w416 -> [_ w428]
                      tunnel: w407 -> [_ w427]
                      frame False {
                      }
                      frame True {
                        n252 = call "获取最近两组水样测试数据.vi"("error in (no error)"=w428, "运行模式"=w427, "table"="叶绿素a") -> ("error out"=w432:errorcluster, "存储变量"=w431:T16)  [unwired: 7 in]
                        n253 = call "集成干预测试数据存储.vi"("error in (no error)"=w432, "存储变量"=w431) -> ("error out"=w429:errorcluster)  [unwired: 9 in]
                      }
                    }
                    n254 = global read "断电保存变量.vi" "藻密度"() -> (w408:bool)
                    n255 = case shown="真" w408 {
                      tunnel: [_ w423] -> _
                      tunnel: w415 -> [_ w422]
                      tunnel: w407 -> [_ w421]
                      frame False {
                      }
                      frame True {
                        n256 = call "获取最近两组水样测试数据.vi"("error in (no error)"=w422, "运行模式"=w421, "table"="藻密度") -> ("error out"=w426:errorcluster, "存储变量"=w425:T16)  [unwired: 7 in]
                        n257 = call "集成干预测试数据存储.vi"("error in (no error)"=w426, "存储变量"=w425) -> ("error out"=w423:errorcluster)  [unwired: 9 in]
                      }
                    }
                  }
                }
              }
            }
          }
        }
        n258 = global read "采配水全局变量.vi" "状态"() -> (w298:T9)
        n259 = Unbundle By Name(w298) -> ("R0"=w297:i16)
        n260 = Equal To 0?(x=w297) -> (x = 0?=w296:bool)
        n261 = Select(t=enum16{"初始化", "采配水启动", "仪器操作", "反冲洗", "结束"}."结束" ("枚举"), s=w296, f=enum16{"初始化", "采配水启动", "仪器操作", "反冲洗", "结束"}."反冲洗" ("枚举")) -> (s? t:f=w293:enum16{"初始化", "采配水启动", "仪器操作", "反冲洗", "结束"})
      }
      frame "结束" {
        n262 = Unbundle By Name(w478) -> ("测试模式"=w479:enum16{"正常测试", "集成干预"})
        n263 = Cancel Notification(0:w481) -> (8:w482:refnum<notifier>)  [unwired: 1 in, 2 out]
        n264 = case shown="\"集成干预\"" w479 {
          tunnel: w477 -> [_ w485]
          frame "正常测试", Default {
          }
          frame "集成干预" {
            n265 = global write "系统设置全局变量.vi" "运行模式"(w485) -> ()
          }
        }
        n266 = Release Notifier(notifier=w482) -> ()  [unwired: 2 in, 3 out]
        n267 = Enqueue Element At Opposite End(queue=w475, element=T2 {"命令"="单个写入", {"starting address"=302, "holding register value"=0}} ("元素")) -> (queue out=w474:refnum<queue>)  [unwired: 2 in, 2 out]
        n268 = Release Queue(queue=w474) -> ()  [unwired: 2 in, 3 out]
      }
    }
    n269 = Format Into String(format string="%s,当前运行时间%d秒" ("格式字符串"), w15, w11) -> (resulting string=w16:string)  [unwired: 2 in, 1 out]
    n270 = global write "采配水全局变量.vi" "运行状态显示"(w16) -> ()
  }
